vi "Destructor.vi"(8 "error in (no error)":errorcluster, 11 "FAMM in":refnum<class "FAMM.lvclass">) -> (0 "error out":errorcluster, 3 "FAMM out":refnum<class "FAMM.lvclass">)   [LabVIEW 2020, in "Sgraph_lib_V1.lvlib" / "FAMM.lvclass"]
doc: "Close the application"
uses:
  FAMM.lvclass
  FAMM.lvclass/FAMM.ctl
  DBAL/controls/DBAL_Command.ctl
  DBAL/controls/DBAL-commands.ctl
  PAQ-memory.lvclass
  DBAL/DBAL.lvclass
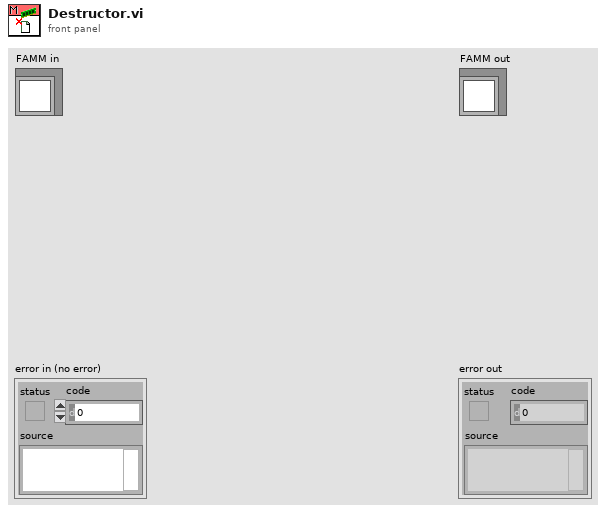
[diagram p1: front panel]
types:
  T1 = typedef "Sgraph_lib_V1.lvlib/DBAL.lvclass/DBAL-commands.ctl" = enum16{"idle", "SavePAQdata", "ExitService"}
  T2 = typedef "Sgraph_lib_V1.lvlib/DBAL.lvclass/DBAL_Command.ctl" = cluster{"Source":string, "Command":T1, "Time Stamp":timestamp, "data":variant}
  T3 = typedef "Sgraph_lib_V1.lvlib/FAMM.lvclass/FAMM-attributes.ctl" = cluster{"FAMM_PAQ_Layers":i32, "FAMM_PAQ_resolution":dbl, "PAQ_TAGs":string[], "WAQ_TAGs":string[], "EAQ_TAGs":string[], "All_TAGs":string[], "PAQtagProps":T4[], "WAQtagProps":T4[], "EAQtagProps":T4[], "DBAL_class":refnum<data-value>, "PAQ_memory":refnum<data-value>[], "PAQupdates":timestamp[], "FAMM_Size":cluster{"other":i32, "1day":i32, "1week":i32}, "DatabaseFileExtention":string, "DatabaseSaveRate":dbl, "Database_path":path, "DBAL-Queue":refnum<queue>, "OS_name":string}
  T4 = typedef "Sgraph_lib_V1.lvlib/typedef_com_TagProp.ctl" = cluster{"Description":string, "EngUnits":string, "RangeH":dbl, "RangeL":dbl, "Resolution":i32, "Obsolete":bool, "ChangeDate":timestamp, "ChangeSource":string, "ChangeReason":string, "TagFunc":u32}
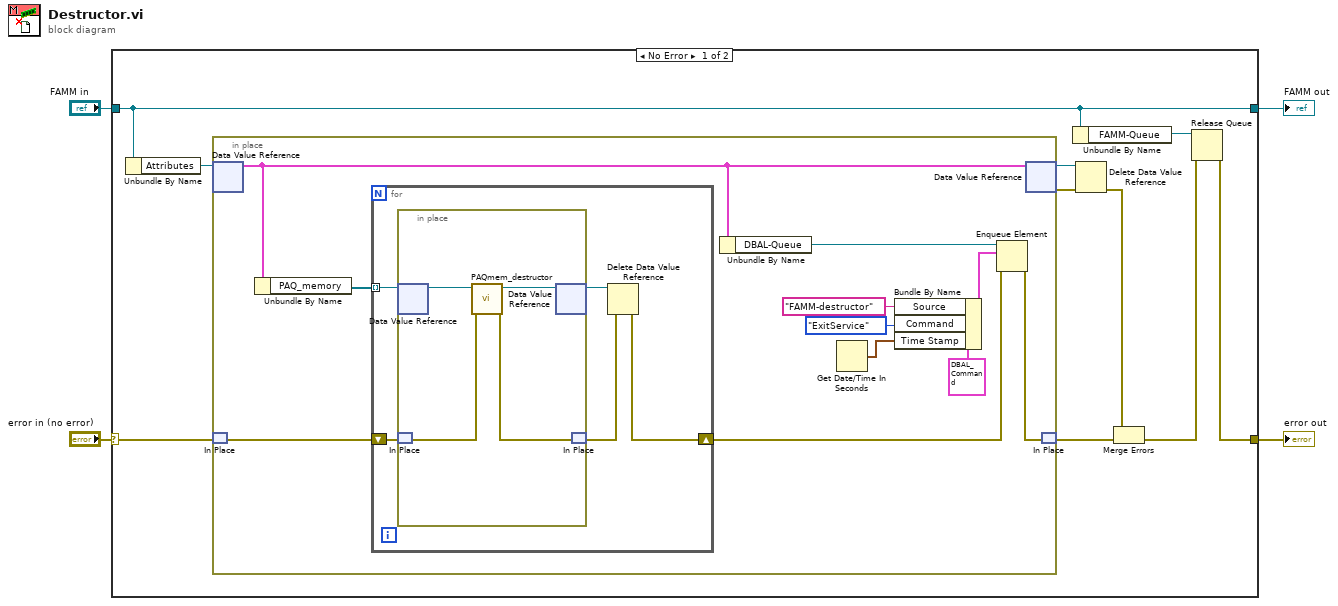
[diagram p0: block diagram]
diagram:
  n1 = case shown="No Error" "error in (no error)" {
    selector: "error in (no error)" -> [w14 w36]
    tunnel: [w5 w36] -> w3
    tunnel: [w8 w35] -> w1
    tunnel: "FAMM in" -> [w8 w35]
    frame No Error {
      n2 = Unbundle By Name(w8) -> ("Attributes"=w9:refnum<data-value>)
      n3 = in-place {
        n4 = in-place-dvr #1(w9) -> (w23:T3)  [unwired: 1 out]
        n5 = in-place-match #2(w14) -> (w24:errorcluster)
        n6 = Unbundle By Name(w23) -> ("PAQ_memory"=w25:refnum<data-value>[])
        n7 = for {
          tunnel: w25 -> [w30] mode=indexing
          shift-right: [w26] -> w19
          shift-left: w24 -> [w29]
          n8 = in-place {
            n9 = in-place-dvr #3(w30) -> (w32:refnum<class "PAQ-memory.lvclass">)  [unwired: 1 out]
            n10 = in-place-match #4(w29) -> (w34:errorcluster)
            n11 = call "PAQmem_destructor.vi"("error in (no error)"=w34, "PAQ-memory in"=w32) -> ("error out"=w33:errorcluster, "PAQ-memory out"=w31:refnum<class "PAQ-memory.lvclass">)  [unwired: 8 in]
            n12 = in-place-dvr #3(w31) -> (w28:refnum<data-value>)  [unwired: 1 out]
            n13 = in-place-match #4(w33) -> (w27:errorcluster)
          }
          n14 = Delete Data Value Reference(data value reference=w28, error in=w27) -> (error out=w26:errorcluster)  [unwired: 1 out]
        }
        n15 = Unbundle By Name(w23) -> ("DBAL-Queue"=w22:refnum<queue>)
        n16 = Get Date/Time In Seconds() -> (seconds since 1Jan1904=w15:timestamp)
        n17 = Bundle By Name(cluster=T2 {"Source"="", "Command"=enum."idle", "Time Stamp"=timestamp(0 s since 1904-01-01), "data"=variant} ("element"), "Source"="FAMM-destructor", "Command"=DBAL-commands."ExitService", "Time Stamp"=w15) -> (w20:T2)
        n18 = Enqueue Element(queue=w22, element=w20, error in (no error)=w19) -> (error out=w18:errorcluster)  [unwired: 1 in, 2 out]
        n19 = in-place-dvr #1(w23) -> (w13:refnum<data-value>, w12:errorcluster)
        n20 = in-place-match #2(w18) -> (w10:errorcluster)
      }
      n21 = Unbundle By Name(w8) -> ("FAMM-Queue"=w7:refnum<queue>)
      n22 = Delete Data Value Reference(data value reference=w13, error in=w12) -> (error out=w11:errorcluster)  [unwired: 1 out]
      n23 = Merge Errors(w11, w10) -> (w6:errorcluster)
      n24 = Release Queue(queue=w7, error in (no error)=w6) -> (error out=w5:errorcluster)  [unwired: 1 in, 2 out]
    }
    frame Error {
    }
  }
  "error out" <- w3
  "FAMM out" <- w1
